vi "InstrParam.vi"(4 "queue out":refnum<queue>, 6 "user event out":refnum<user-event>, 8 "error in (no error)":errorcluster caption="entrée d'erreur (pas d'erreur)", 10 "InstrParam":string, 11 "AppliedMotionDrive en entrée":refnum<class "AppliedMotionDrive.lvclass"> caption="DNL_LabVIEW Object in") -> (0 "error out":errorcluster caption="sortie d'erreur", 3 "AppliedMotionDrive en sortie":refnum<class "AppliedMotionDrive.lvclass"> caption="DNL_LabVIEW Object out")   [LabVIEW 2019, in "AppliedMotionDrive.lvclass"]
uses:
  AppliedMotionDrive.lvclass
  C:/Programmes Labview/LabscanV1A/DevicesClass/BaseDevice/BaseDevice.lvclass
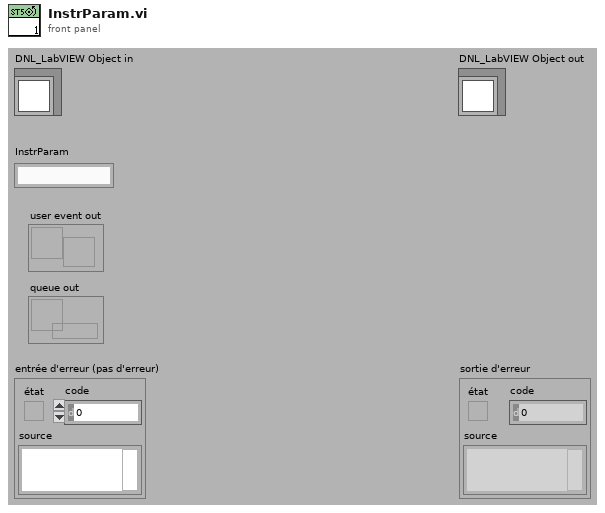
[diagram p1: front panel]
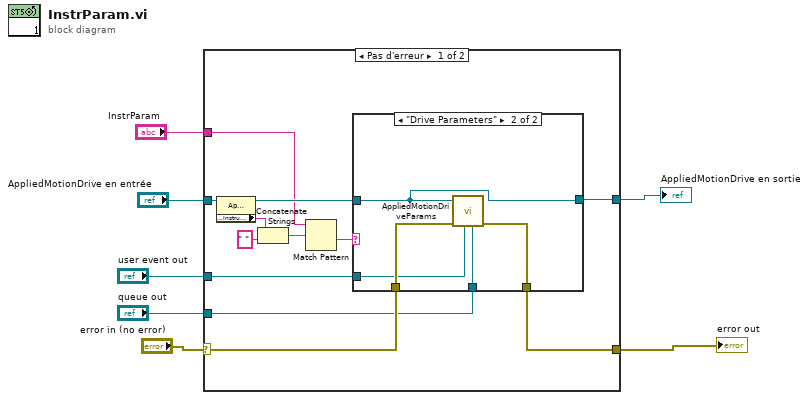
[diagram p0: block diagram]
diagram:
  n1 = case shown="Pas d'erreur" "error in (no error)" {
    selector: "error in (no error)" -> [w19 w28]
    tunnel: [w18 w28] -> w6
    tunnel: "InstrParam" -> [w13 _]
    tunnel: "AppliedMotionDrive en entrée" -> [w16 w27]
    tunnel: [w17 w27] -> w3
    tunnel: "user event out" -> [w9 _]
    tunnel: "queue out" -> [w8 _]
    frame No Error {
      n2 = property class="AppliedMotionDrive.lvclass"(reference=w16) -> (reference out=w15:refnum<class "AppliedMotionDrive.lvclass">, "Accessor:InstrumentName"=w14:string)  [unwired: 1 in, 1 out]
      n3 = Concatenate Strings(w14, " " ("chaîne")) -> (w12:string)
      n4 = Match Pattern(string=w13, regular expression=w12) -> (after substring=w10:string)  [unwired: 1 in, 3 out]
      n5 = case shown="\"Drive Parameters\"" w10 {
        tunnel: w15 -> [w21 w22]
        tunnel: w19 -> [w20 w26]
        tunnel: [w20 w25] -> w18
        tunnel: [w21 w22] -> w17
        tunnel: w9 -> [_ w24]
        tunnel: w8 -> [_ w23]
        frame Default {
        }
        frame "Drive Parameters" {
          n6 = call "AppliedMotionDriveParams.vi"("queue out"=w23, "user event out"=w24, "error in (no error)"=w26, "AppliedMotionDrive.lvclass"=w22) -> ("error out"=w25:errorcluster)  [unwired: 6 in, 1 out]
        }
      }
    }
    frame Error {
    }
  }
  "error out" <- w6
  "AppliedMotionDrive en sortie" <- w3
